vi "Data_Execution.vi"(6 "Queues":T2, 8 "Status/Errors in":refnum<vi>, 10 "Process data parameters in":T4={"Stop loop"={"Settings changed?"=FALSE, "Stop?"=refnum}, "Button refs"={"Stop program"=refnum, "Save settings"=refnum, "DAQ mode"=refnum, "Reset settings"=refnum, "Apply settings"=refnum, "Reset MAS"=refnum, "Reset SLV"=refnum, "Local DBase?"=refnum, "Last value DBase"=FALSE, "Database"=refnum, "Calibration"=refnum, "Save settings 2"=refnum}, "Process messages"={"Process message mode"=enum."Error", "Slave data?"=FALSE, "Length get settings message"=0, "Delta time"=0.0, "Data_Filter"={"Filter_Data"=FALSE, "Use_Thresh"=FALSE, "Reduce data?"=FALSE}, "Time_difference_stack"=[], "Starting sec"=0, "Ending sec"=0, "Ending sec 2"=0, "MAS_Page_Thresh"=refnum, "SLV_Page_Thresh"=refnum, "Database"=refnum}, "Settings state"={"MAS locked?"=refnum, "SLV locked?"=refnum}, "Mode"={"Mode"=enum."Dialog", "Expert?"=FALSE, "Dialog?"=FALSE}, "Alignment parameters"=refnum, "Timer parameters"=refnum, "Files"={"Path config file"=path "", "Path def. ini file"=path "", "Path ini file 1"=path "", "Path ini file 2"=path "", "Path RBF file"=path ""}, "Time difference"=refnum, "Alignment"={"GEN_Page_Calibrate"=refnum, "MAS_Page_Gain"=refnum, "MAS_Page_Offset"=refnum, "SLV_Page_Gain"=refnum, "SLV_Page_Offset"=refnum, "MAS_Page_Common"=refnum, "SLV_Page_Common"=refnum}, "Page Statistics"=refnum}, 11 "Devices in":T1) -> (0 "Status/Errors out":refnum<vi>, 2 "Process data parameters out":T4={"Stop loop"={"Settings changed?"=FALSE, "Stop?"=refnum}, "Button refs"={"Stop program"=refnum, "Save settings"=refnum, "DAQ mode"=refnum, "Reset settings"=refnum, "Apply settings"=refnum, "Reset MAS"=refnum, "Reset SLV"=refnum, "Local DBase?"=refnum, "Last value DBase"=FALSE, "Database"=refnum, "Calibration"=refnum, "Save settings 2"=refnum}, "Process messages"={"Process message mode"=enum."Error", "Slave data?"=FALSE, "Length get settings message"=0, "Delta time"=0.0, "Data_Filter"={"Filter_Data"=FALSE, "Use_Thresh"=FALSE, "Reduce data?"=FALSE}, "Time_difference_stack"=[], "Starting sec"=0, "Ending sec"=0, "Ending sec 2"=0, "MAS_Page_Thresh"=refnum, "SLV_Page_Thresh"=refnum, "Database"=refnum}, "Settings state"={"MAS locked?"=refnum, "SLV locked?"=refnum}, "Mode"={"Mode"=enum."Dialog", "Expert?"=FALSE, "Dialog?"=FALSE}, "Alignment parameters"=refnum, "Timer parameters"=refnum, "Files"={"Path config file"=path "", "Path def. ini file"=path "", "Path ini file 1"=path "", "Path ini file 2"=path "", "Path RBF file"=path ""}, "Time difference"=refnum, "Alignment"={"GEN_Page_Calibrate"=refnum, "MAS_Page_Gain"=refnum, "MAS_Page_Offset"=refnum, "SLV_Page_Gain"=refnum, "SLV_Page_Offset"=refnum, "MAS_Page_Common"=refnum, "SLV_Page_Common"=refnum}, "Page Statistics"=refnum}, 3 "Devices out":T1, 4 "Command":T3)   [LabVIEW 2013]
uses:
  Controls/Process_Data_Parameters.ctl
  Controls/Stop_Loop.ctl
  Controls/Button_Refs.ctl
  Controls/Process_Messages.ctl
  Controls/Process_Message_Mode.ctl
  Controls/Settings_State.ctl
  Controls/Mode.ctl
  Controls/Files.ctl
  Controls/Page_Calibration.ctl
  Controls/Command_Process_Messages.ctl
  Controls/Queues.ctl
  Controls/One_Second.ctl
  Controls/GPS_Timestamp.ctl
  Controls/Devices.ctl
  Controls/Device_Elements.ctl
  Controls/Get_Set_Device_Options.ctl
  Controls/Get_Set_Settings_State_Options.ctl
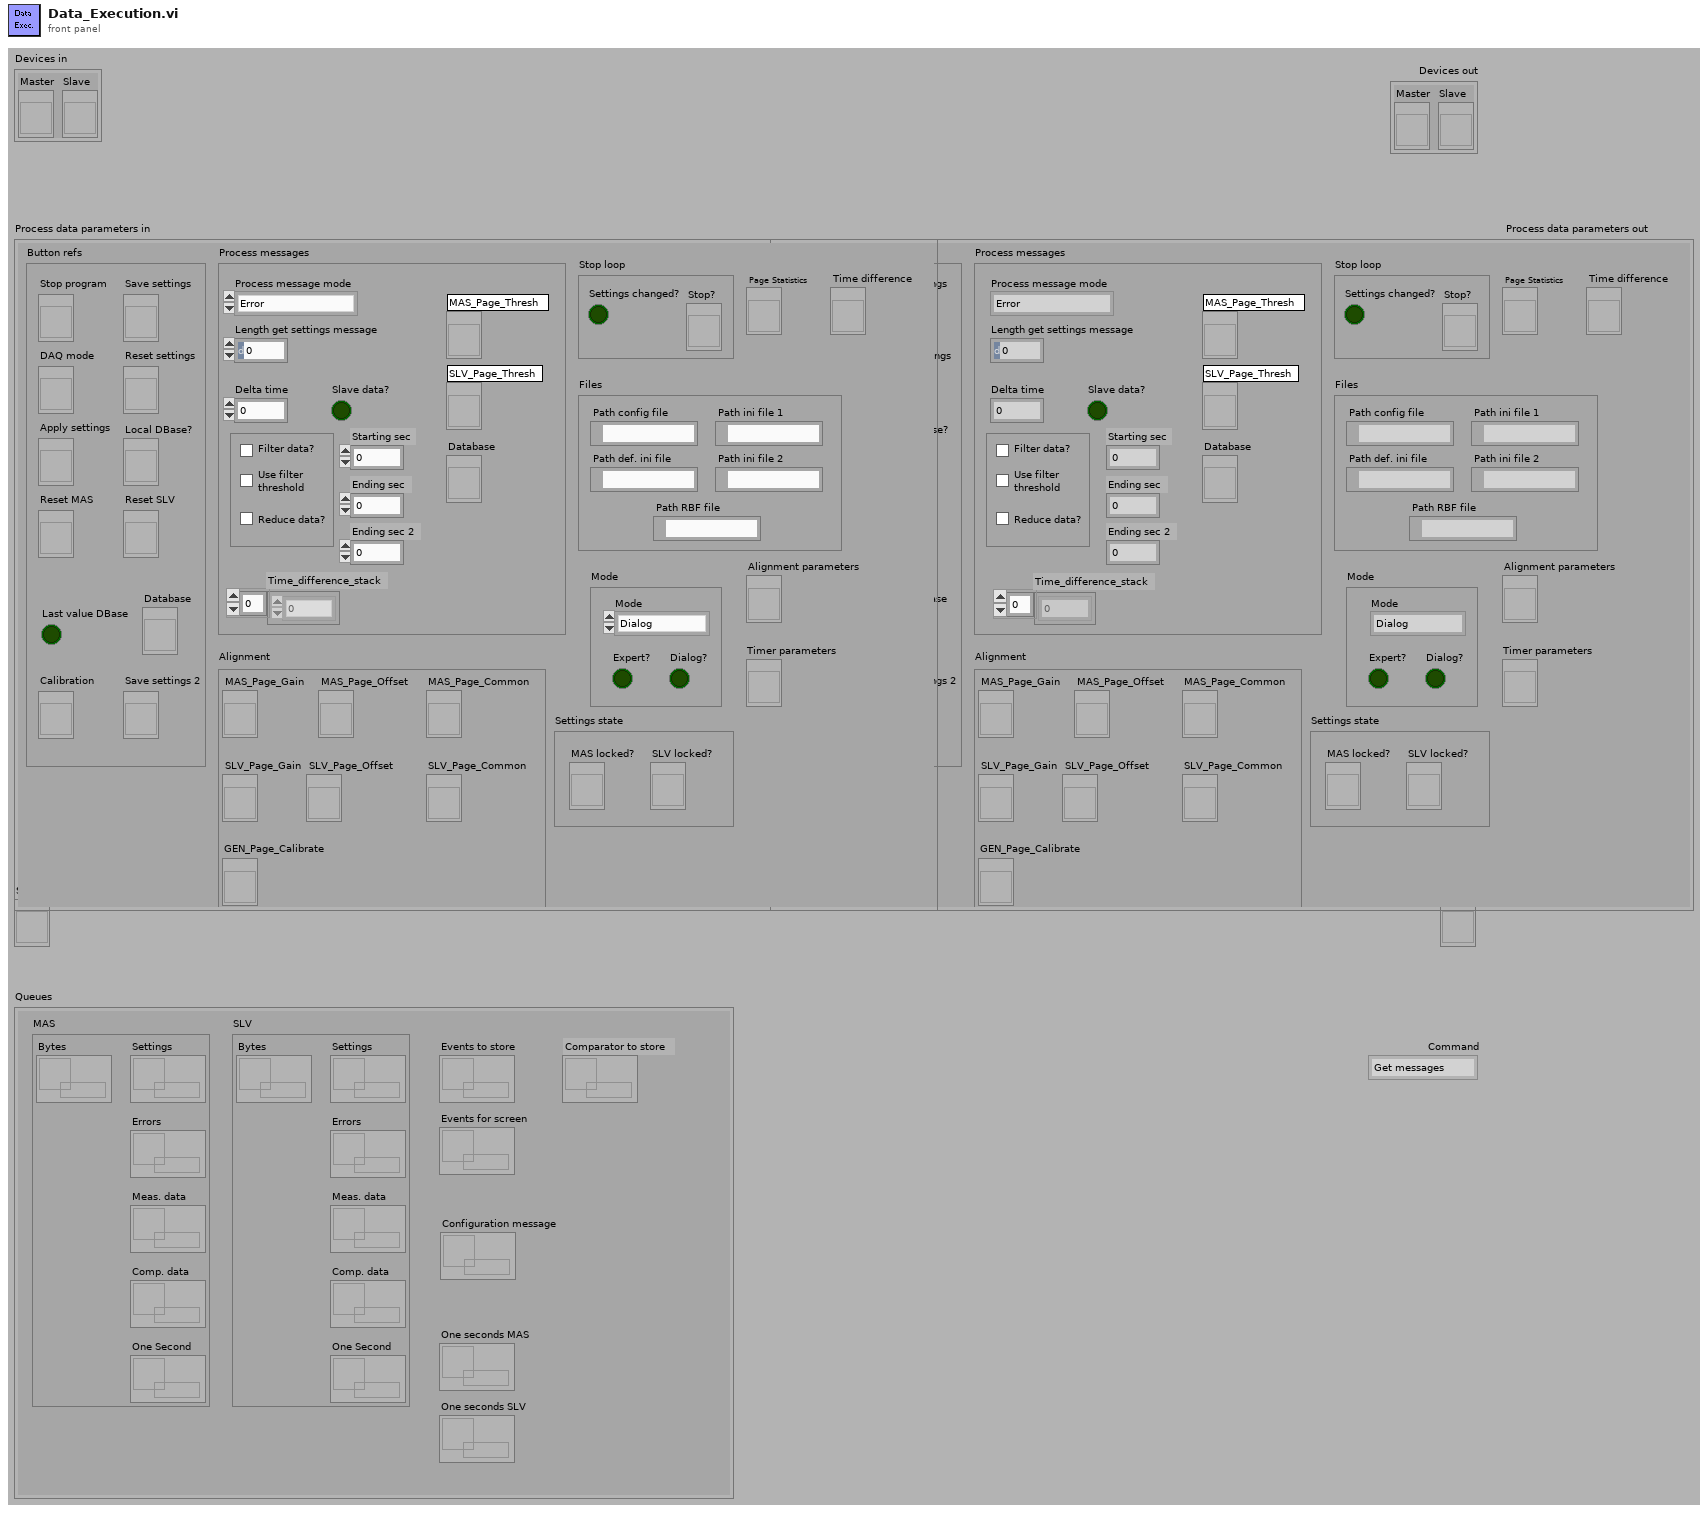
[diagram p1: front panel]
types:
  T1 = typedef "Devices.ctl" = cluster{"Master":refnum<vi>, "Slave":refnum<vi>}
  T2 = typedef "Queues.ctl" = cluster{"MAS":cluster{"Bytes":refnum<queue>, "Settings":refnum<queue>, "Errors":refnum<queue>, "Meas. data":refnum<queue>, "One Second":refnum<queue>, "Comp. data":refnum<queue>}, "SLV":cluster{"Bytes":refnum<queue>, "Settings":refnum<queue>, "Errors":refnum<queue>, "Meas. data":refnum<queue>, "One Second":refnum<queue>, "Comp. data":refnum<queue>}, "Events to store":refnum<queue>, "Events for screen":refnum<queue>, "One seconds MAS":refnum<queue>, "One seconds SLV":refnum<queue>, "Configuration message":refnum<queue>, "Comparator to store":refnum<queue>}
  T3 = typedef "Command_Process_Messages.ctl" = enum16{"Get messages", "Process messages", "Stop loop", "No action"}
  T4 = typedef "Process_Data_Parameters.ctl" = cluster{"Stop loop":T5, "Button refs":T6, "Process messages":T7, "Settings state":T9, "Mode":T10, "Alignment parameters":refnum<vi>, "Timer parameters":refnum<vi>, "Files":T11, "Time difference":refnum<vi>, "Alignment":T12, "Page Statistics":refnum<vi>}
  T5 = typedef "Stop_Loop.ctl" = cluster{"Settings changed?":bool, "Stop?":refnum<vi>}
  T6 = typedef "Button_Refs.ctl" = cluster{"Stop program":refnum<vi>, "Save settings":refnum<vi>, "DAQ mode":refnum<vi>, "Reset settings":refnum<vi>, "Apply settings":refnum<vi>, "Reset MAS":refnum<vi>, "Reset SLV":refnum<vi>, "Local DBase?":refnum<vi>, "Last value DBase":bool, "Database":refnum<vi>, "Calibration":refnum<vi>, "Save settings 2":refnum<vi>}
  T7 = typedef "Process_Messages.ctl" = cluster{"Process message mode":T8, "Slave data?":bool, "Length get settings message":i32, "Delta time":dbl, "Data_Filter":cluster{"Filter_Data":bool, "Use_Thresh":bool, "Reduce data?":bool}, "Time_difference_stack":u64[], "Starting sec":u64, "Ending sec":u64, "Ending sec 2":u64, "MAS_Page_Thresh":refnum<vi>, "SLV_Page_Thresh":refnum<vi>, "Database":refnum<vi>}
  T8 = typedef "Process_Message_Mode.ctl" = enum16{"Error", "Measurement data", "Comparator data", "One Second"}
  T9 = typedef "Settings_State.ctl" = cluster{"MAS locked?":refnum<vi>, "SLV locked?":refnum<vi>}
  T10 = typedef "Mode.ctl" = cluster{"Mode":enum8{"Stop", "Dialog", "Hisparc II", "Hisparc II DAQ", "Alignment"}, "Expert?":bool, "Dialog?":bool}
  T11 = typedef "Files.ctl" = cluster{"Path config file":path, "Path def. ini file":path, "Path ini file 1":path, "Path ini file 2":path, "Path RBF file":path}
  T12 = typedef "Page_Calibration.ctl" = cluster{"GEN_Page_Calibrate":refnum<vi>, "MAS_Page_Gain":refnum<vi>, "MAS_Page_Offset":refnum<vi>, "SLV_Page_Gain":refnum<vi>, "SLV_Page_Offset":refnum<vi>, "MAS_Page_Common":refnum<vi>, "SLV_Page_Common":refnum<vi>}
  T13 = typedef "Get_Set_Settings_State_Options.ctl" = enum16{"Get", "Lock", "Unlock"}
  T14 = typedef "Get_Set_Device_Options.ctl" = enum16{"Get", "Get cluster", "Set"}
  T15 = typedef "Device_Elements.ctl" = enum16{"Default", "Master?", "Connected?", "Status", "Disconnect?", "Handle", "Version number"}
  T16 = typedef "Device.ctl" = cluster{"Master?":T17, "Connected?":bool, "Status":bool, "Disconnect?":bool, "Handle":u32, "Version number":u32}
  T17 = typedef "Master.ctl" = enum16{"Master", "Slave", "General"}
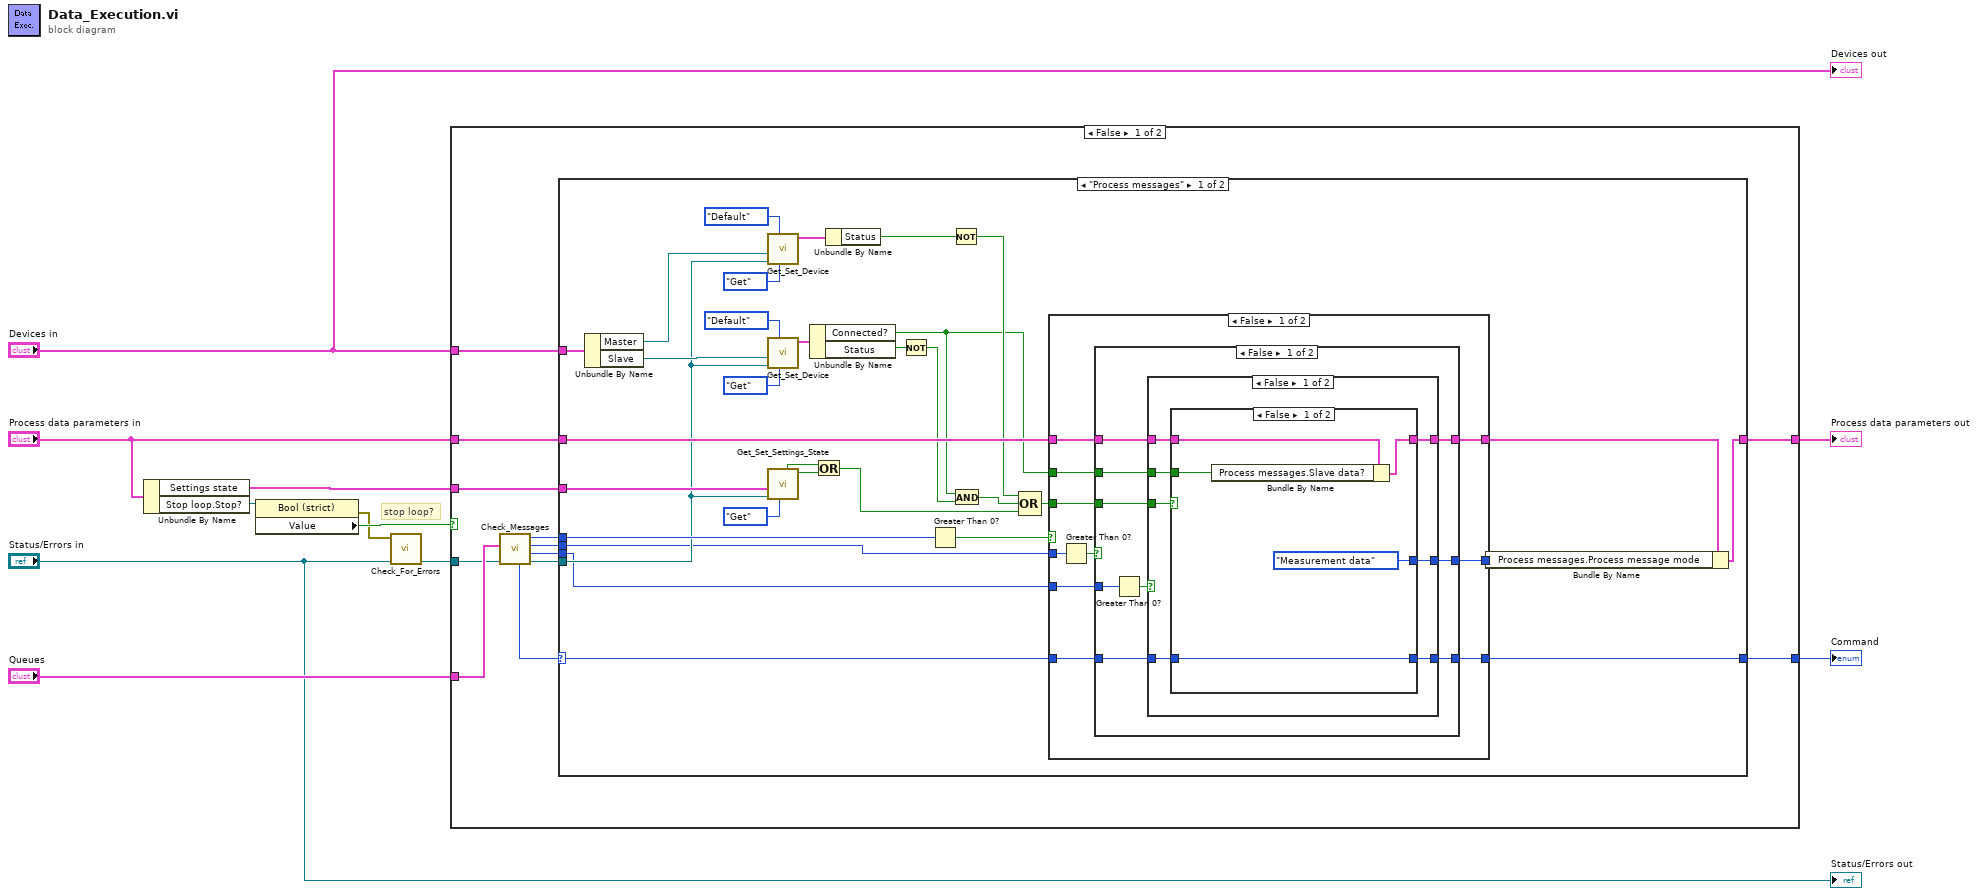
[diagram p0: block diagram]
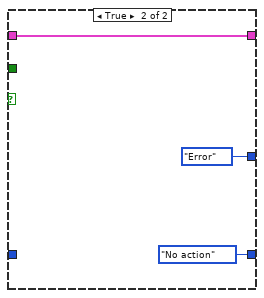
[diagram p2: hidden frame]
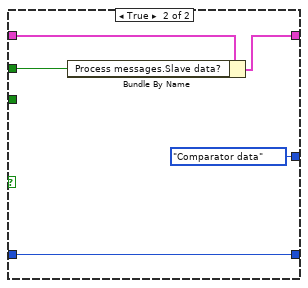
[diagram p3: hidden frame]
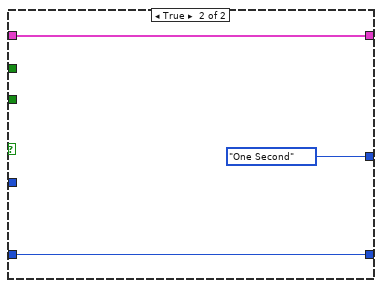
[diagram p4: hidden frame]
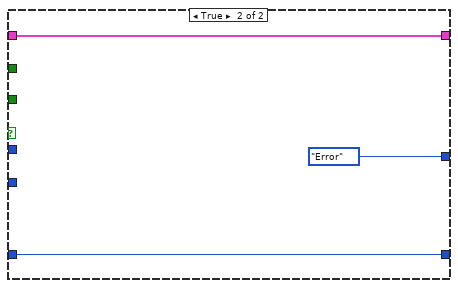
[diagram p5: hidden frame]
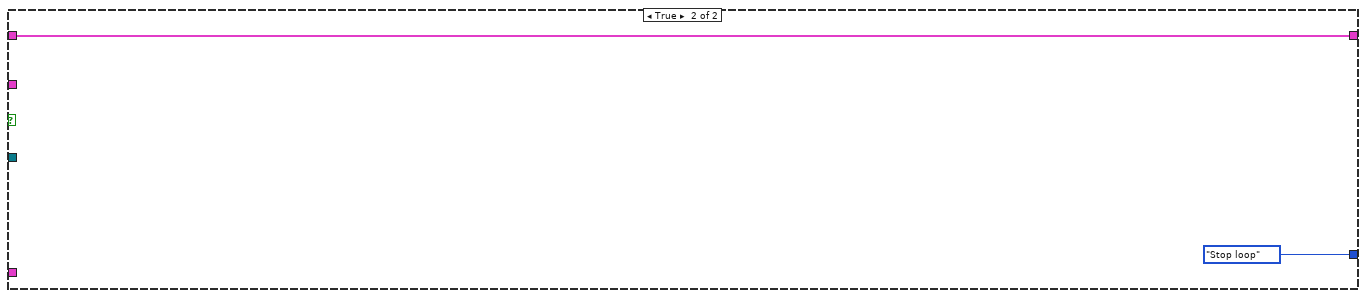
[diagram p7: hidden frame]
diagram:
  # "stop loop?"
  n1 = Unbundle By Name("Process data parameters in") -> ("Settings state"=w1:T9, "Stop loop.Stop?"=w7:refnum<vi>)
  n2 = property class="Bool (strict)"(reference=w7) -> (error out=w2:errorcluster, "Value"=w5:bool)  [unwired: 1 in, 1 out]
  n3 = call "Check_For_Errors.vi"("Status/Errors in"="Status/Errors in", "error in"=w2) -> ("Status/Errors out"=w3:refnum<vi>)  [unwired: 9 out]
  n4 = case shown="False" w5 {
    tunnel: "Queues" -> [w22 _]
    tunnel: w3 -> [w18 _]
    tunnel: "Process data parameters in" -> [w21 w103]
    tunnel: "Devices in" -> [w17 _]
    tunnel: [w20 w103] -> w9
    tunnel: [w19 Command_Process_Messages."Stop loop" ("Command")] -> w8
    tunnel: w1 -> [w15 _]
    frame False {
      n5 = call "Check_Messages.vi"("Status/Errors in"=w18, "Queues"=w22) -> ("Status/Errors out"=w16:refnum<vi>, "# Comparator data"=w12:i32, "# One Second"=w13:i32, "# errors"=w23:i32, "Get/process"=w14:T3)  [unwired: 1 in, 4 out]
      n6 = case shown="\"Process messages\"" w14 {
        selector: w14 -> [w40 w102]
        tunnel: [w41 w102] -> w19
        tunnel: w23 -> [w50 _]
        tunnel: w21 -> [w53 w101]
        tunnel: [w55 w101] -> w20
        tunnel: w17 -> [w43 _]
        tunnel: w16 -> [w35 _]
        tunnel: w15 -> [w42 _]
        tunnel: w13 -> [w25 _]
        tunnel: w12 -> [w24 _]
        frame "Process messages" {
          n7 = Unbundle By Name(w43) -> ("Master"=w36:refnum<vi>, "Slave"=w47:refnum<vi>)
          n8 = call "Get_Set_Device.vi"("Get/Set"=Get_Set_Device_Options."Get", "Element"=Device_Elements."Default", "Status/Errors in"=w35, "Device in"=w36) -> ("Device"=w39:T16)  [unwired: 1 in, 6 out]
          n9 = call "Get_Set_Device.vi"("Get/Set"=Get_Set_Device_Options."Get", "Element"=Device_Elements."Default", "Status/Errors in"=w35, "Device in"=w47) -> ("Device"=w46:T16)  [unwired: 1 in, 6 out]
          n10 = call "Get_Set_Settings_State.vi"("Get/Set"=Get_Set_Settings_State_Options."Get", "Status/Errors in"=w35, "Settings state"=w42) -> ("SLV locked?"=w49:bool, "MAS locked?"=w48:bool)  [unwired: 2 in, 5 out]
          n11 = Unbundle By Name(w46) -> ("Connected?"=w27:bool, "Status"=w28:bool)
          n12 = Or(x=w48, y=w49) -> (x .or. y?=w33:bool)
          n13 = Unbundle By Name(w39) -> ("Status"=w32:bool)
          n14 = Not(x=w28) -> (.not. x?=w26:bool)
          n15 = Greater Than 0?(x=w50) -> (x > 0?=w54:bool)
          n16 = Not(x=w32) -> (.not. x?=w31:bool)
          n17 = And(x=w27, y=w26) -> (x .and. y?=w29:bool)
          n18 = Compound Arithmetic op=OR(w31, w29, w33) -> (w34:bool)
          n19 = case shown="False" w54 {
            tunnel: w25 -> [w61 _]
            tunnel: [w65 Process_Message_Mode."Error" ("Process messages.Process message mode")] -> w51
            tunnel: w53 -> [w64 w99]
            tunnel: [w63 w99] -> w52
            tunnel: w27 -> [w62 _]
            tunnel: w34 -> [w59 _]
            tunnel: [w58 w98] -> w41
            tunnel: w40 -> [w57 w98]
            tunnel: w24 -> [w56 _]
            frame False {
              n20 = Greater Than 0?(x=w61) -> (x > 0?=w60:bool)
              n21 = case shown="False" w60 {
                tunnel: [w74 Process_Message_Mode."One Second" ("Process messages.Process message mode")] -> w65
                tunnel: w64 -> [w73 w96]
                tunnel: [w66 w96] -> w63
                tunnel: w62 -> [w72 _]
                tunnel: w59 -> [w71 _]
                tunnel: [w70 w95] -> w58
                tunnel: w57 -> [w69 w95]
                tunnel: w56 -> [w68 _]
                frame False {
                  n22 = Greater Than 0?(x=w68) -> (x > 0?=w67:bool)
                  n23 = case shown="False" w67 {
                    tunnel: [w77 Process_Message_Mode."Comparator data" ("Process messages.Process message mode")] -> w74
                    tunnel: w73 -> [w81 w92]
                    tunnel: [w76 w91] -> w66
                    tunnel: w72 -> [w80 w90]
                    tunnel: w71 -> [w79 _]
                    tunnel: [w78 w94] -> w70
                    tunnel: w69 -> [w75 w94]
                    frame False {
                      n24 = case shown="False" w79 {
                        tunnel: [Process_Message_Mode."Measurement data" ("Process messages.Process message mode") Process_Message_Mode."Error" ("Process messages.Process message mode")] -> w77
                        tunnel: w81 -> [w85 w87]
                        tunnel: [w84 w87] -> w76
                        tunnel: w80 -> [w83 _]
                        tunnel: [w82 Command_Process_Messages."No action" ("Command")] -> w78
                        tunnel: w75 -> [w82 _]
                        frame False {
                          n25 = Bundle By Name(cluster=w85, "Process messages.Slave data?"=w83) -> (w84:T4)
                        }
                        frame True {
                        }
                      }
                    }
                    frame True {
                      n26 = Bundle By Name(cluster=w92, "Process messages.Slave data?"=w90) -> (w91:T4)
                    }
                  }
                }
                frame True {
                }
              }
            }
            frame True {
            }
          }
          n27 = Bundle By Name(cluster=w52, "Process messages.Process message mode"=w51) -> (w55:T4)
        }
        frame Default {
        }
      }
    }
    frame True {
    }
  }
  "Process data parameters out" <- w9
  "Command" <- w8
  "Status/Errors out" <- "Status/Errors in"
  "Devices out" <- "Devices in"
